vi "Stop RFSG.vi"(0 "Path in":refnum<class "Scalar Path.lvclass">, 11 "error in (no error)":errorcluster) -> (4 "Path out":refnum<class "Scalar Path.lvclass">, 15 "error out":errorcluster)   [LabVIEW 2023, in "RFFixtureCharact.Public.lvlib" / "Scalar Path.lvclass"]
uses:
  Scalar Path.lvclass
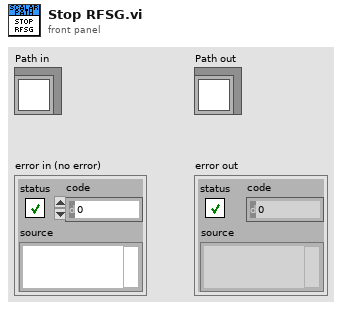
[diagram p1: front panel]
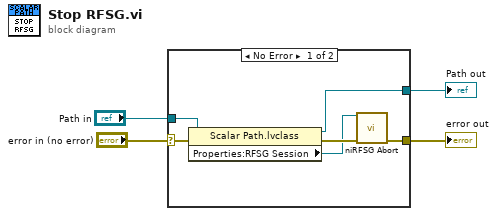
[diagram p0: block diagram]
diagram:
  n1 = case shown="No Error" "error in (no error)" {
    selector: "error in (no error)" -> [w9 w12]
    tunnel: [w6 w12] -> w3
    tunnel: [w8 w11] -> w2
    tunnel: "Path in" -> [w10 w11]
    frame No Error {
      n2 = property class="Scalar Path.lvclass"(reference=w10, error in=w9) -> (reference out=w8:refnum<class "Scalar Path.lvclass">, error out=w7:errorcluster, "Properties:RFSG Session"=w5:refnum<k15>)
      n3 = call <instrlib>:"niRFSG Abort.vi"("instrument handle"=w5, "error in"=w7) -> ("error out"=w6:errorcluster)  [unwired: 12 in, 1 out]
    }
    frame Error {
    }
  }
  "error out" <- w3
  "Path out" <- w2
